vi "Start Module.vi"(8 "error in":errorcluster) -> (0 "error out":errorcluster)   [LabVIEW 2020, in "SECS Bridge.lvlib"]
uses:
  SECS Bridge.lvlib
  Private/SECS Bridge Main.vi
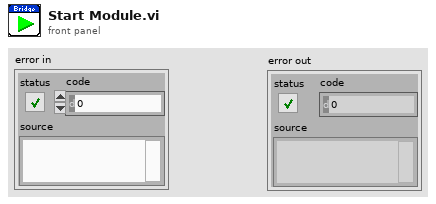
[diagram p1: front panel]
types:
  T1 = enum32{"Bad", "Idle", "Run top level", "Running"}
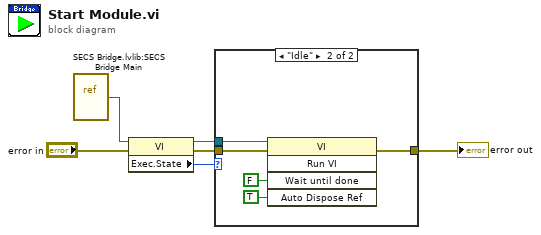
[diagram p0: block diagram]
diagram:
  n1 = vi-ref "SECS Bridge.lvlib:SECS Bridge Main.vi"() -> (w6:refnum<vi>)
  n2 = property class="VI"(reference=w6, error in="error in") -> (reference out=w2:refnum<vi>, error out=w3:errorcluster, "Exec.State"=w4:T1)
  n3 = case shown="\"Idle\"" w4 {
    tunnel: w3 -> [w7 w12]
    tunnel: w2 -> [_ w11]
    tunnel: [w7 w10] -> w1
    frame "Bad", Default {
    }
    frame "Idle" {
      n4 = invoke class="VI" method="Run VI"(reference=w11, error in=w12, "Wait until done"=FALSE ("Wait Until Done"), "Auto Dispose Ref"=TRUE ("Auto Dispose Reference")) -> (error out=w10:errorcluster)  [unwired: 1 in, 4 out]
    }
  }
  "error out" <- w1
